vi "Select - Select Between 2 Numeric Values Using a Boolean Button.vi"() -> ()   [LabVIEW 2016]
panel:
  out "s ? t:f":dbl
  in  "s":bool
  in  "f":dbl
  in  "t":dbl
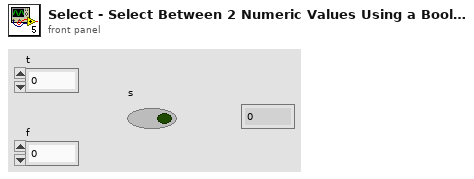
[diagram p1: front panel]
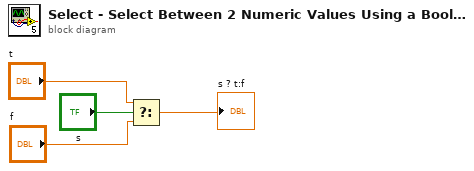
[diagram p0: block diagram]
diagram:
  n1 = Select(t="t", s="s", f="f") -> (s? t:f=→"s ? t:f":dbl)
